vi "[Test] Create directory.vi"() -> ()   [LabVIEW 2015, in "Tests.lvlib"]
uses:
  Tests.lvlib
  Protocol.ctl
  classes/File Transfer Behavior/File Transfer Behavior.lvclass
panel:
  in  "Password":string
  in  "Username":string
  in  "Protocol":T1
  in  "Address":string
  in  "Path":string
  out "error out":errorcluster
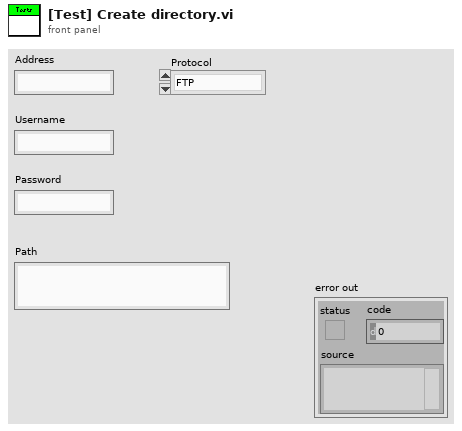
[diagram p1: front panel]
types:
  T1 = typedef "Tests.lvlib/Protocol.ctl" = enum16{"FTP", "WebDAV"}
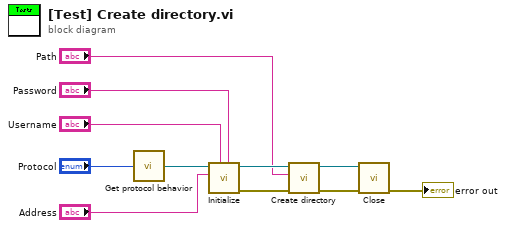
[diagram p0: block diagram]
diagram:
  n1 = call "Get protocol behavior.vi"("Protocol"="Protocol") -> ("RT Management.lvlib:FTP.lvclass"=w11:refnum<class "File Transfer Behavior.lvclass">)
  n2 = call-dynamic "Initialize.vi"("Password"="Password", "Username"="Username", "Address"="Address", "File Transfer Behavior in"=w11) -> ("error out"=w10:errorcluster, "File Transfer Behavior out"=w9:refnum<class "File Transfer Behavior.lvclass">)  [unwired: 6 in]
  n3 = call-dynamic "Create directory.vi"("error in (no error)"=w10, "Directory"="Path", "File Transfer Behavior in"=w9) -> ("error out"=w8:errorcluster, "File Transfer Behavior out"=w7:refnum<class "File Transfer Behavior.lvclass">)  [unwired: 7 in]
  n4 = call-dynamic "Close.vi"("error in (no error)"=w8, "File Transfer Behavior in"=w7) -> ("error out"=→"error out":errorcluster)  [unwired: 9 in]
